vi "Read Status Byte Register.vi"(8 "error in (no error)":errorcluster, 11 "VISA resource name":refnum<visa-resource-name>) -> (0 "error out":errorcluster, 1 "Event Summary Bit":bool, 2 "Message Available Bit":bool, 3 "VISA resource name out":refnum<visa-resource-name>, 4 "Status Byte Register Cluster":T1, 5 "Status Byte Register":i32)   [LabVIEW 2014, in "Associated Research SC6540.lvlib"]
doc: "Read the Status Byte from the instrument."
uses:
  <instrlib>/Associated Research SC6540/Associated Research SC6540.lvlib
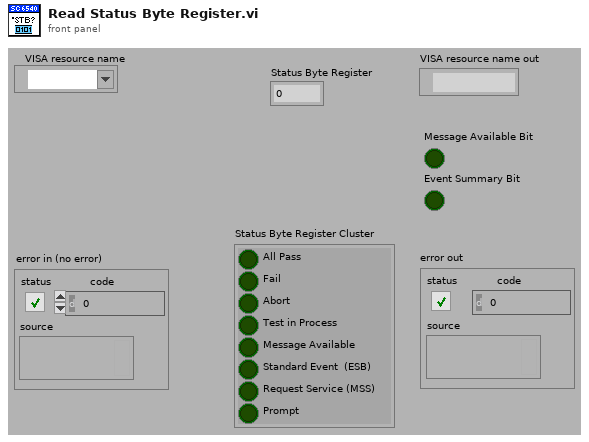
[diagram p1: front panel]
types:
  T1 = cluster{"All Pass":bool, "Fail":bool, "Abort":bool, "Test in Process":bool, "Message Available":bool, "Standard Event  (ESB)":bool, "Request Service (MSS)":bool, "Prompt":bool}
  T2 = cluster{"Boolean array[0]":bool, "Boolean array[1]":bool, "Boolean array[2]":bool, "Boolean array[3]":bool, "Boolean array[4]":bool, "Boolean array[5]":bool, "Boolean array[6]":bool, "Boolean array[7]":bool}
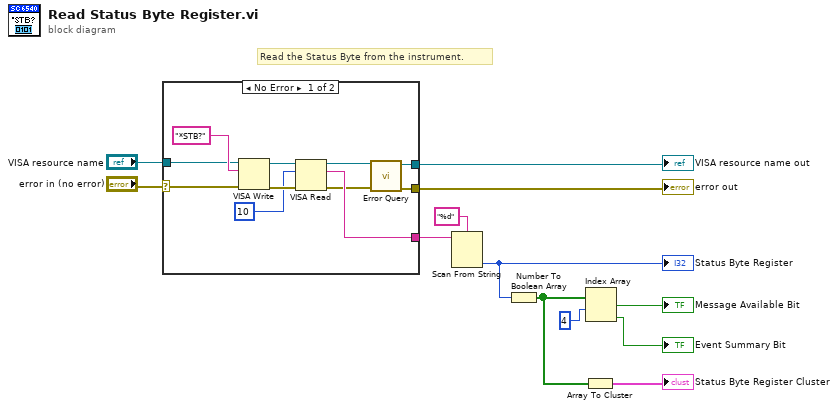
[diagram p0: block diagram]
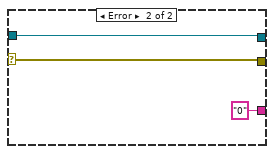
[diagram p2: hidden frame]
diagram:
  # "Read the Status Byte from the instrument."
  n1 = case shown="No Error" "error in (no error)" {
    selector: "error in (no error)" -> [w23 w25]
    tunnel: "VISA resource name" -> [w19 w26]
    tunnel: [w17 "0" ("read buffer")] -> w4
    tunnel: [w14 w26] -> w2
    tunnel: [w13 w25] -> w1
    frame No Error {
      n2 = VISA Write(VISA resource name=w19, write buffer="*STB?" ("Command to Send (empty)"), error in (no error)=w23) -> (VISA resource name out=w21:refnum<visa-resource-name>, error out=w22:errorcluster)  [unwired: 1 out]
      n3 = VISA Read(VISA resource name=w21, byte count=u32 10, error in (no error)=w22) -> (VISA resource name out=w16:refnum<visa-resource-name>, read buffer=w17:string, error out=w15:errorcluster)  [unwired: 1 out]
      n4 = call <instrlib>:"Error Query.vi"("error in (no error)"=w15, "VISA resource name"=w16) -> ("error out"=w13:errorcluster, "VISA resource name out"=w14:refnum<visa-resource-name>)  [unwired: 6 in, 2 out]
    }
    frame Error {
    }
  }
  "error out" <- w1
  "VISA resource name out" <- w2
  n5 = Scan From String(format string="%d" ("Format String"), input string=w4) -> (output 1=w10:i32)  [unwired: 3 in, 3 out]
  "Status Byte Register" <- w10
  n6 = Number To Boolean Array(number=w10) -> (Boolean array=w7:bool[])
  n7 = Array To Cluster(array=w7) -> (cluster=→"Status Byte Register Cluster":T2)
  n8 = Index Array(array=w7, index #1=4 ("Index")) -> (element #1=→"Message Available Bit":bool, element #2=→"Event Summary Bit":bool)  [unwired: 1 in]
